vi "Sensor.vi"(8 "error in (no error)":errorcluster) -> (0 "error out":errorcluster)   [LabVIEW 2017]
uses:
  Type Definitions/Queue FG Options.ctl
panel:
  in  "Funds dispensed":bool
  in  "Deposit received":bool
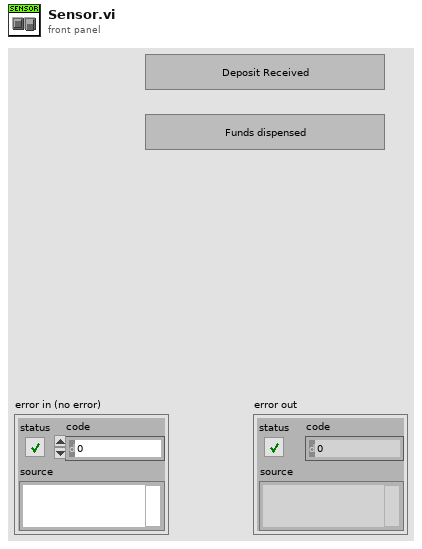
[diagram p1: front panel]
types:
  T1 = typedef "Queue FG Options.ctl" = enum16{"Set", "Get", "Read", "Write", "Destroy"}
  T2 = typedef "Sensor States.ctl" = enum16{"Shutdown", "Initial", "Idle"}
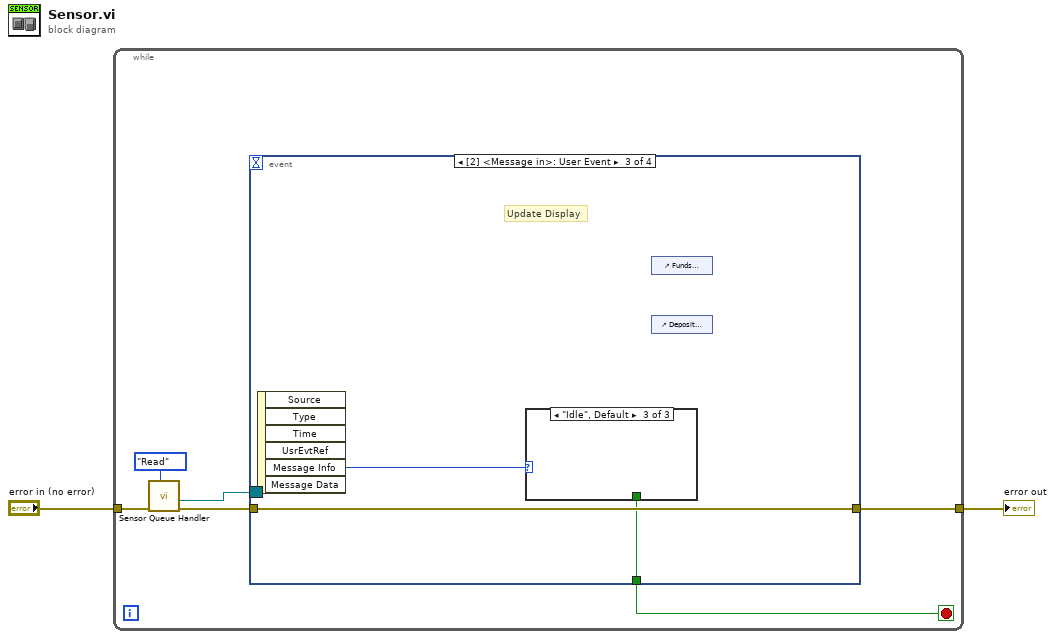
[diagram p0: block diagram]
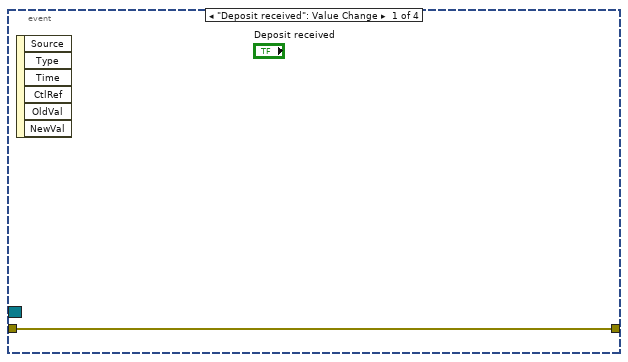
[diagram p2: hidden frame]
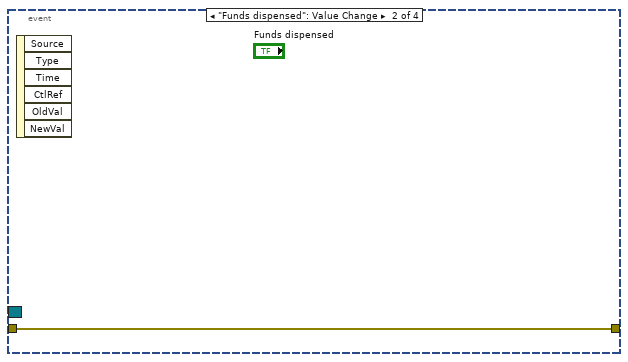
[diagram p3: hidden frame]
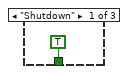
[diagram p4: hidden frame]
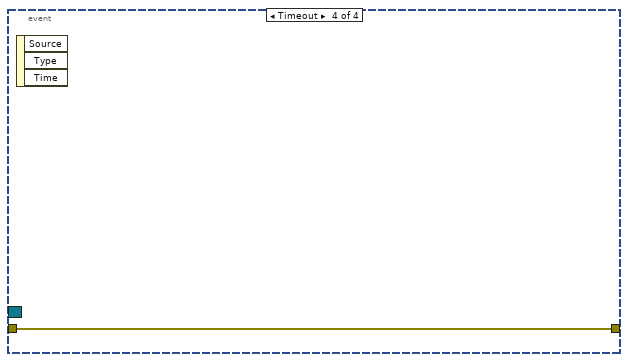
[diagram p6: hidden frame]
diagram:
  n1 = while {
    tunnel: "error in (no error)" -> [w7]
    tunnel: [w5] -> w1
    stop <- w3 stop-if-true
    n2 = call "Sensor Queue Handler.vi"("Action"=Queue_FG_Options."Read", "error in (no error)"=w7) -> ("error out"=w6:errorcluster, "Event Registration Refnum"=w4:refnum<event-registration>)  [unwired: 6 in, 2 out]
    n3 = event shown="[2] <Message in>: User Event" {
      selector: w4 -> [_ _ _ _]
      dyn-events: _ -> [_ _ _ _]
      timeout: _ -> [_ _ _ _]
      tunnel: w6 -> [w9 w10 w13 w15]
      tunnel: [w9 w10 w13 w15] -> w5
      tunnel: [_ _ w11 _] -> w3
      event "Deposit received": Value Change {
        n4 = event-data() -> ()  [unwired: 1 in, 6 out]
      }
      event "Funds dispensed": Value Change {
        n5 = event-data() -> ()  [unwired: 1 in, 6 out]
      }
      event User Event {
        # "Update Display"
        n6 = event-data() -> ("Message Info"=w12:T2)  [unwired: 1 in, 5 out]
        n7 = case shown="\"Idle\", Default" w12 {
          tunnel: [TRUE _ _] -> w11
          frame "Shutdown" {
          }
          frame "Initial" {
          }
          frame "Idle", Default {
          }
        }
        n8 = control-ref of="Funds dispensed"() -> ()  [unwired: 1 out]
        n9 = control-ref of="Deposit received"() -> ()  [unwired: 1 out]
      }
      event Timeout {
        n10 = event-data() -> ()  [unwired: 1 in, 3 out]
      }
    }
  }
  "error out" <- w1
